vi "Set Target - Check & Resend.vi"(8 "error in (no error)":errorcluster, 11 "Mercury Targets":T1) -> (0 "error out":errorcluster, 3 "Magnet = Target":bool)   [LabVIEW 2016, in "IPS-120-API.lvlib"]
uses:
  IPS-120-API.lvlib
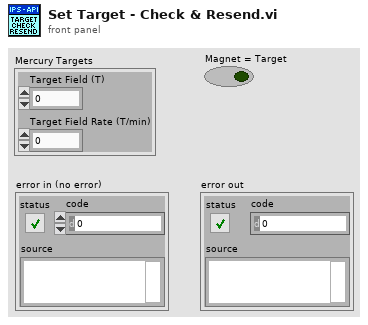
[diagram p1: front panel]
types:
  T1 = cluster{"Target Field (T)":dbl, "Target Field Rate (T/min)":dbl}
  T2 = cluster{"Hold":bool, "Clamp":bool, "To Set":bool, "To Zero":bool, "Send to IPS":bool, "PS Heat":bool}
  T3 = cluster{"Magnet Field":dbl, "PS Field":dbl, "Target Field":dbl, "Target Field Rate":dbl, "Voltage":dbl, "Current":dbl, "Switch":bool}
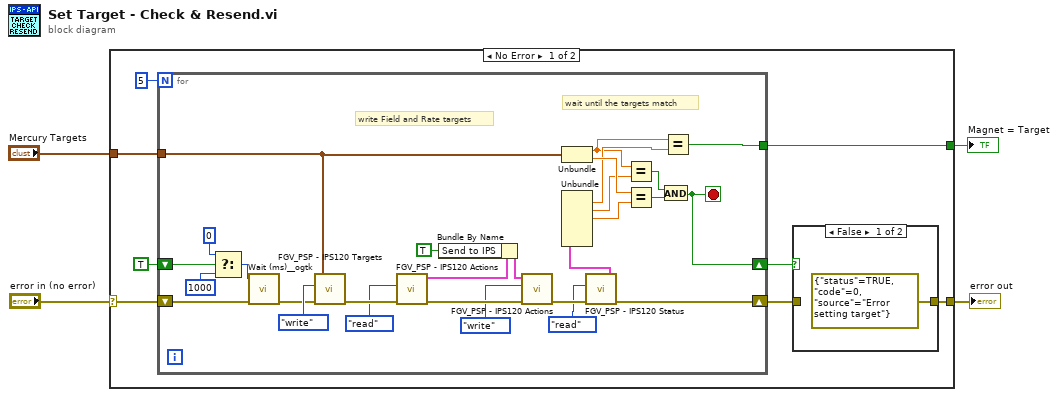
[diagram p0: block diagram]
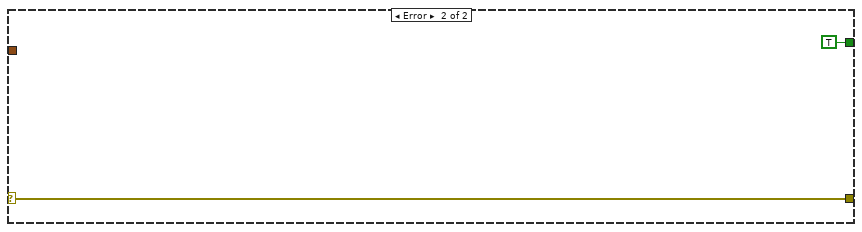
[diagram p3: hidden frame]
diagram:
  n1 = case shown="No Error" "error in (no error)" {
    selector: "error in (no error)" -> [w5 w44]
    tunnel: [w12 TRUE] -> w4
    tunnel: "Mercury Targets" -> [w11 _]
    tunnel: [w7 w44] -> w2
    frame No Error {
      n2 = for {
        N: 5 -> [_]
        tunnel: [w38] -> w12
        tunnel: w11 -> [w33]
        shift-right: [w37] -> w8
        shift-left: w5 -> [w21]
        shift-right: [w23] -> w9
        shift-left: TRUE -> [w19]
        stop <- w23 stop-if-true
        # "wait until the targets match"
        # "write Field and Rate targets"
        n3 = Select(t=u32 0 ("milliseconds to wait"), s=w19, f=u32 1000 ("milliseconds to wait")) -> (s? t:f=w16:u32)
        n4 = call <userlib>:"Wait (ms)__ogtk.vi"("error in (no error)"=w21, "milliseconds to wait"=w16) -> ("error out"=w20:errorcluster)  [unwired: 8 in, 1 out]
        n5 = call "FGV_PSP - IPS120 Targets.vi"("error in"=w20, "Function"=enum16{"write", "read"}."write", "Targets"=w33) -> ("error out"=w39:errorcluster)  [unwired: 3 in, 1 out]
        n6 = call "FGV_PSP - IPS120 Actions.vi"("error in"=w39, "Function"=enum16{"write", "read"}."read") -> ("error out"=w41:errorcluster, "actions"=w40:T2)  [unwired: 4 in]
        n7 = Bundle By Name(cluster=w40, "Send to IPS"=TRUE) -> (w42:T2)
        n8 = call "FGV_PSP - IPS120 Actions.vi"("error in"=w41, "Function"=enum16{"write", "read"}."write", "actions"=w42) -> ("error out"=w34:errorcluster)  [unwired: 3 in, 1 out]
        n9 = Unbundle(w33) -> ("Target Field (T)"=w24:dbl, "Target Field Rate (T/min)"=w32:dbl)
        n10 = call "FGV_PSP - IPS120 Status.vi"("error in"=w34, "Function"=enum16{"write", "read"}."read") -> ("error out"=w37:errorcluster, "status"=w27:T3)  [unwired: 4 in]
        n11 = Unbundle(w27) -> ("PS Field"=w25:dbl, "Target Field"=w28:dbl, "Target Field Rate"=w29:dbl)  [unwired: 4 out]
        n12 = Equal?(x=w24, y=w28) -> (x = y?=w26:bool)
        n13 = Equal?(x=w32, y=w29) -> (x = y?=w30:bool)
        n14 = And(x=w26, y=w30) -> (x .and. y?=w23:bool)
        n15 = Equal?(x=w24, y=w25) -> (x = y?=w38:bool)
      }
      n16 = case shown="False" w9 {
        tunnel: w8 -> [_ w14]
        tunnel: [errorcluster {"status"=TRUE, "code"=0, "source"="Error setting target"} ("error in (no error)") w14] -> w7
        frame False {
        }
        frame True {
        }
      }
    }
    frame Error {
    }
  }
  "Magnet = Target" <- w4
  "error out" <- w2
